vi "Binary Subtraction.vi"(10 "NUM 2 (Binary)":i32 format="%b", 11 "NUM 1 (Binary)":i32 format="%b") -> (3 "Difference  (Binary)":i32 format="%b")   [LabVIEW 2020]
doc: "This VI will find the difference between two Binary Numbers."
panel:
  # "Note: NUUM 1 > NUM 2"
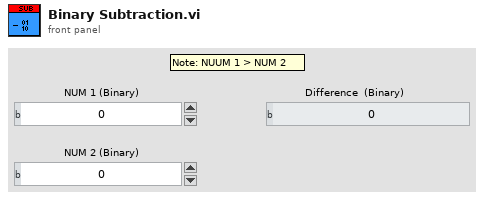
[diagram p1: front panel]
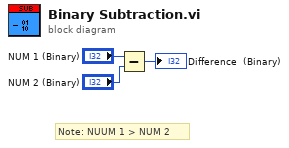
[diagram p0: block diagram]
diagram:
  # "Note: NUUM 1 > NUM 2"
  n1 = Subtract(x="NUM 1 (Binary)", y="NUM 2 (Binary)") -> (x-y=→"Difference  (Binary)":i32)
